vi "MenuTareas.vi"() -> ()   [LabVIEW 2019, in "Aplicacion.lvclass"]
uses:
  Aplicacion.lvclass
  blr_alstom/Controls/Check Cluster.ctl
  blr_alstom/Controls/Configuracion Check Control.ctl
panel:
  out "estadoPrueba1 5":bool
  out "estadoPrueba1 4":bool
  out "estadoPrueba1 3":bool
  in  "estado":enum16{"pendiente", "cumple", "no cumple"}(ring)
  out "estadoPrueba1 2":bool
  out "Arreglo Check Configuracion out":T1
  # "MENU DE PRUEBAS"
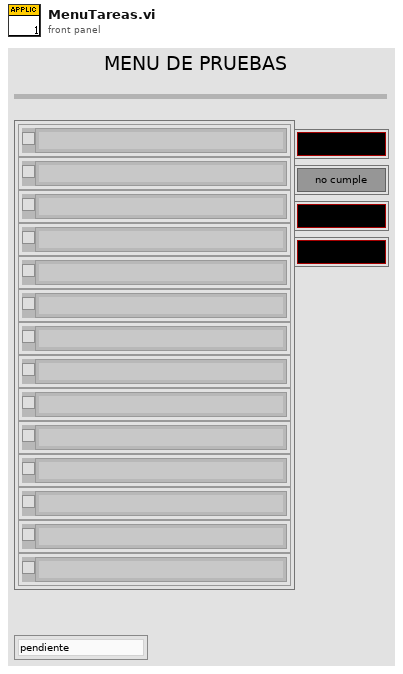
[diagram p1: front panel]
types:
  T1 = typedef "Configuracion Check Control.ctl" = T2[]
  T2 = typedef "Check Cluster.ctl" = cluster{"Check":bool, "Prueba":string}
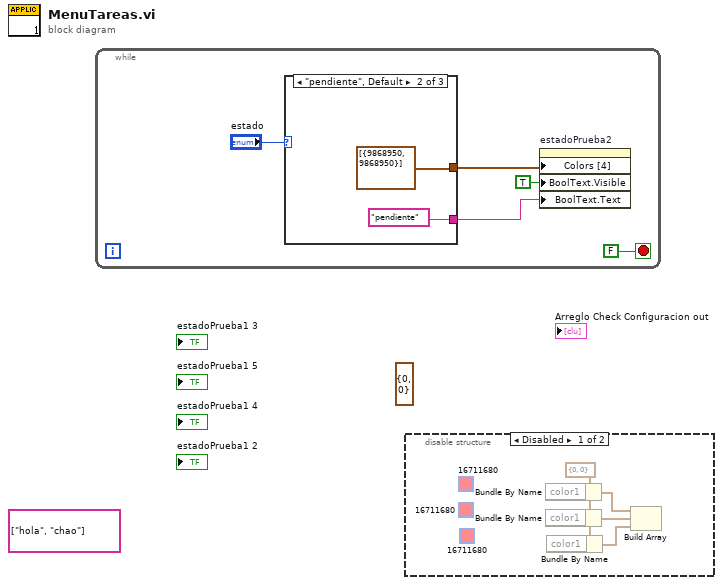
[diagram p0: block diagram]
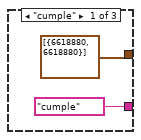
[diagram p3: hidden frame]
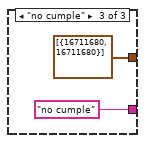
[diagram p4: hidden frame]
diagram:
  (unwired) cluster{"color1":u32, "color2":u32} {"color1"=0, "color2"=0}
  (unwired) string[] ["hola", "chao"] ("Strings [4]")
  n1 = while {
    stop <- FALSE stop-if-true
    n2 = case shown="\"pendiente\", Default" "estado" {
      tunnel: ["cumple" "pendiente" "no cumple"] -> w3
      tunnel: [cluster{u32, u32}[] [{6618880, 6618880}] cluster{u32, u32}[] [{9868950, 9868950}] cluster{u32, u32}[] [{16711680, 16711680}]] -> w1
      frame "cumple" {
      }
      frame "pendiente", Default {
      }
      frame "no cumple" {
      }
    }
    n3 = property on="estadoPrueba2" class="Bool (strict)"("Colors [4]"=w1, "BoolText.Visible"=TRUE ("Boolean Text.Visible"), "BoolText.Text"=w3) -> ()  [unwired: 2 in, 2 out]
  }
  n4 = disable-structure shown="Disabled" {
    frame Disabled {
      (unwired) u32 16711680
      (unwired) u32 16711680
      (unwired) u32 16711680
      w17 = cluster{"color1":u32, "color2":u32} {"color1"=0, "color2"=0}
      n5 = Bundle By Name(cluster=w17) -> (w13:cluster{"color1":u32, "color2":u32}, "color1"=w14:u32)
      n6 = Bundle By Name(cluster=w17) -> (w12:cluster{"color1":u32, "color2":u32}, "color1"=w15:u32)
      n7 = Bundle By Name(cluster=w17) -> (w18:cluster{"color1":u32, "color2":u32}, "color1"=w16:u32)
      n8 = Build Array(w13, w12, w18) -> ()  [unwired: 1 out]
    }
    frame Enabled {
    }
  }
